vi "Reset.vi"(8 "error in (no error)":errorcluster, 10 "Reset Command (0: Reset to Power On)":u16(ring) items=["Reset to Power On", "Reset From Disable"], 11 "VISA resource name":refnum<visa-resource-name>) -> (0 "error out":errorcluster, 3 "VISA resource name out":refnum<visa-resource-name>)   [LabVIEW 2021, in "Sorensen M9A Series.lvlib"]
doc: "This VI resets the Sorensen power supply by sending one of two commands. If the Reset Command terminal is left unwired or wired to 0, the CLR command is sent, which resets the power supply to the Power ON condition. If the Reset Command terminal is wired to 1, the RST command is sent, which resets the power supply to current voltage and current settings if the power supply was disabled by overvoltage or foldback protection."
uses:
  Sorensen M9A Series.lvlib
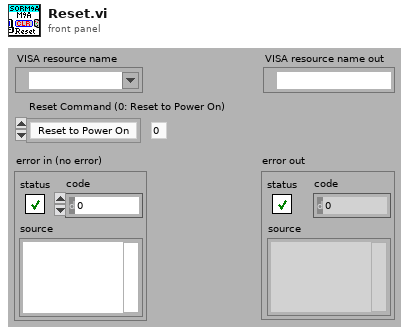
[diagram p1: front panel]
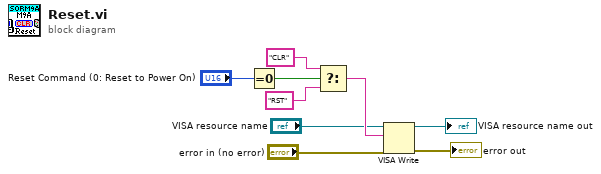
[diagram p0: block diagram]
diagram:
  n1 = Equal To 0?(x="Reset Command (0: Reset to Power On)") -> (x = 0?=w4:bool)
  n2 = Select(t="CLR", s=w4, f="RST") -> (s? t:f=w3:string)
  n3 = VISA Write(VISA resource name="VISA resource name", write buffer=w3, error in (no error)="error in (no error)") -> (VISA resource name out=→"VISA resource name out":refnum<visa-resource-name>, error out=→"error out":errorcluster)  [unwired: 1 out]
